vi "PWD.vi"(8 "error in (no error)":errorcluster, 11 "FTP in":refnum<class "FTP.lvclass">) -> (0 "error out":errorcluster, 2 "Current Directory":string, 3 "FTP out":refnum<class "FTP.lvclass">)   [LabVIEW 2013, in "FTP.lvlib" / "FTP.lvclass"]
uses:
  FTP.lvclass
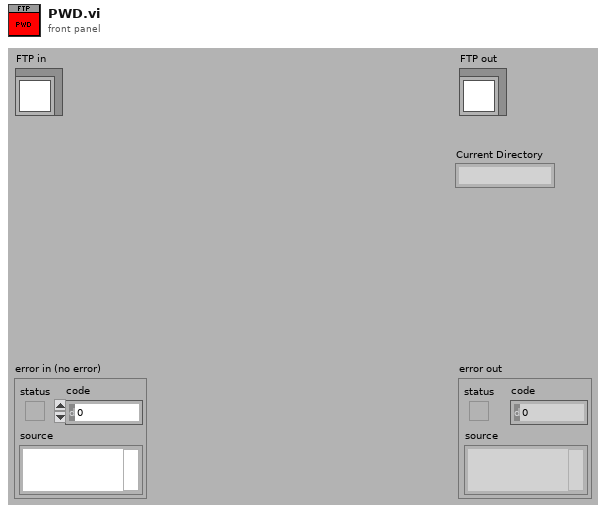
[diagram p1: front panel]
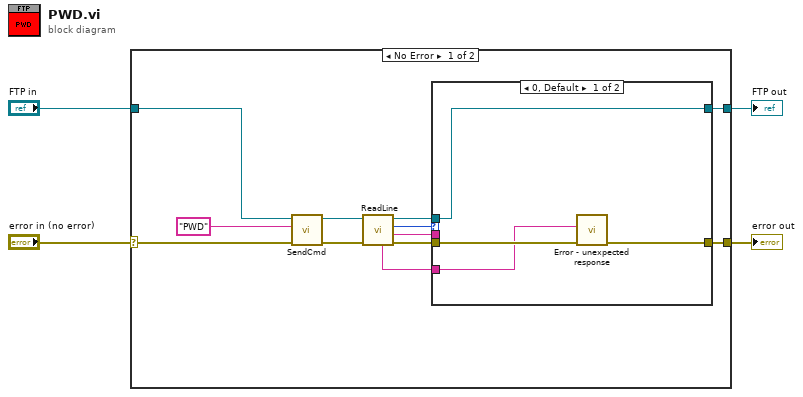
[diagram p0: block diagram]
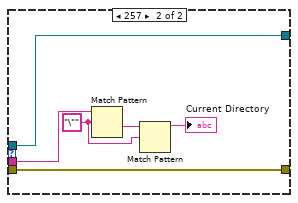
[diagram p2: hidden frame]
diagram:
  n1 = case shown="No Error" "error in (no error)" {
    selector: "error in (no error)" -> [w15 w28]
    tunnel: [w7 w28] -> w3
    tunnel: [w8 w27] -> w1
    tunnel: "FTP in" -> [w16 w27]
    frame No Error {
      n2 = call "SendCmd.vi"("error in (no error)"=w15, "cmd"="PWD", "FTP in"=w16) -> ("error out"=w13:errorcluster, "FTP out"=w14:refnum<class "FTP.lvclass">)  [unwired: 7 in]
      n3 = call "ReadLine.vi"("error in (no error)"=w13, "FTP in"=w14) -> ("error out"=w11:errorcluster, "Line"=w6:string, "code"=w10:i32, "FTP out"=w9:refnum<class "FTP.lvclass">, "Full Line"=w5:string)  [unwired: 5 in]
      n4 = case shown="0, Default" w10 {
        tunnel: w11 -> [w19 w25]
        tunnel: w9 -> [w20 w26]
        tunnel: [w20 w26] -> w8
        tunnel: [w17 w25] -> w7
        tunnel: w6 -> [_ w24]
        tunnel: w5 -> [w18 _]
        frame 0, Default {
          n5 = call "Error - unexpected response.vi"("error in (no error)"=w19, "Full Response"=w18) -> ("error out"=w17:errorcluster)  [unwired: 9 in]
        }
        frame 257 {
          w22 = "\"" ("format string")
          n6 = Match Pattern(string=w24, regular expression=w22) -> (after substring=w23:string)  [unwired: 1 in, 3 out]
          n7 = Match Pattern(string=w23, regular expression=w22) -> (before substring=→"Current Directory":string)  [unwired: 1 in, 3 out]
        }
      }
    }
    frame Error {
    }
  }
  "error out" <- w3
  "FTP out" <- w1
